vi "EventLogger.Task.FlushToDisk.vi"   [LabVIEW 2019, in "Tools.lvlib"]
uses:
  Tools.lvlib
  EventLogger.Task.FlushToDisk.Action.ctl
  CitTemplate/citTemplate.errData.ctl
types:
  T1 = typedef "Tools.lvlib/citTemplate.errData.ctl" = cluster{"action":string, "error":errorcluster}
  T2 = typedef "Tools.lvlib/EventLogger.Task.FlushToDisk.Action.ctl" = enum32{"idle", "constructor", "destructor", "--- EventLogger.Task.FlushToDisk ---"}
  T3 = typedef "Tools.lvlib/citTemplate.notifierHandle.ctl" = refnum<notifier>
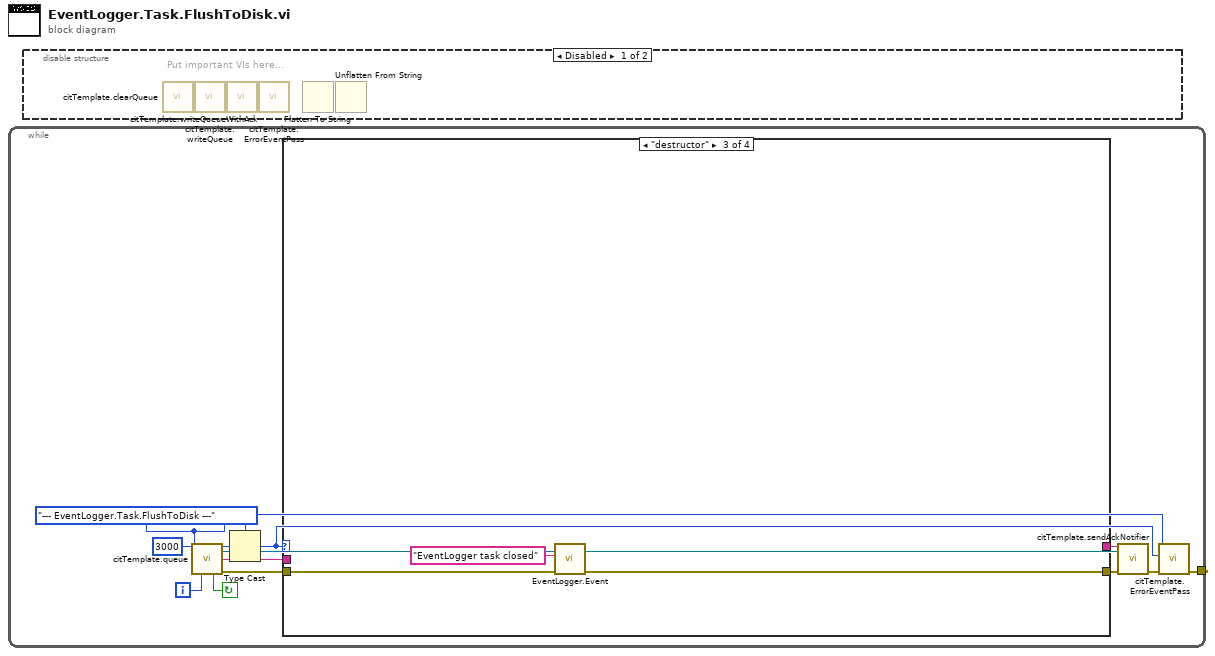
[diagram p0: block diagram]
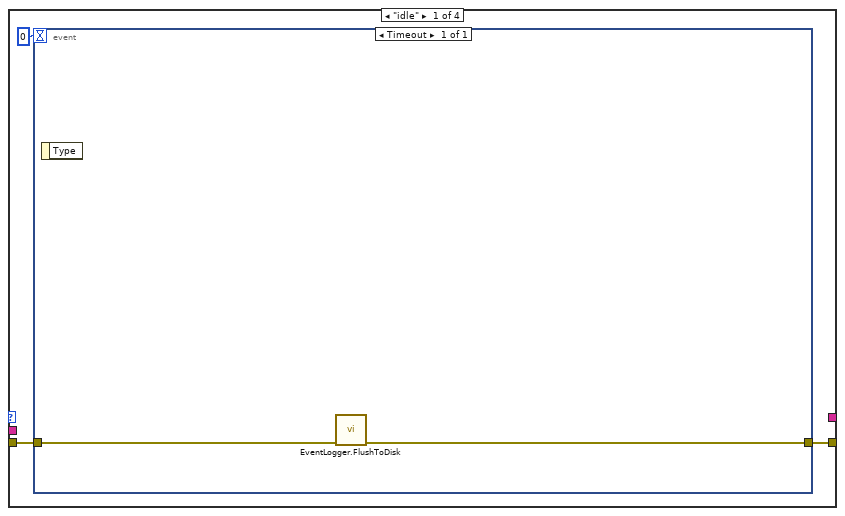
[diagram p3: hidden frame]
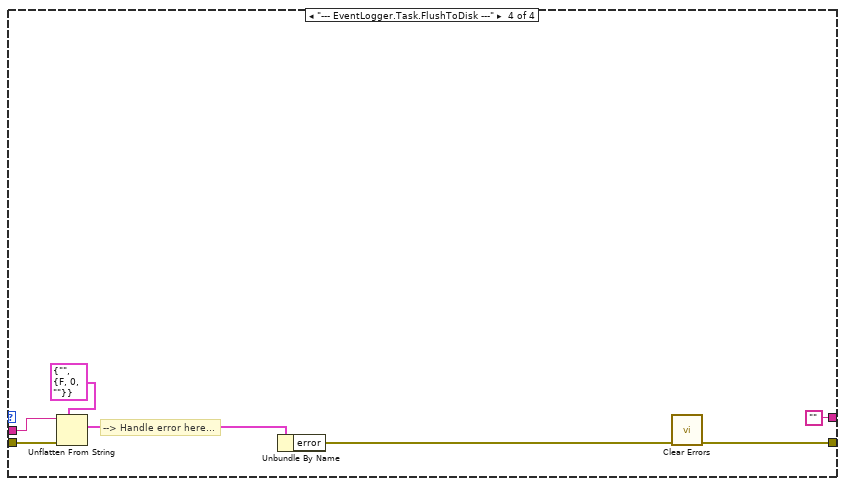
[diagram p5: hidden frame]
diagram:
  n1 = while {
    tunnel: [w2] -> _
    i -> [w8]
    stop <- w9 continue-if-true
    w1 = EventLogger.Task.FlushToDisk.Action."--- EventLogger.Task.FlushToDisk ---" ("Action")
    n2 = call "citTemplate.queue.vi"("ms timeout (250 ms)"=3000, "event enum"=w1, "iteration (-1)"=w8) -> ("notifierHandle out"=w6:T3, "event out"=w12:u32, "(flatten) data out"=w11:string, "continue"=w9:bool, "error out"=w10:errorcluster)  [unwired: 2 in, 6 out]
    n3 = Type Cast(type=w1, x=w12) -> (*(type *) &x=w3:T2)
    n4 = case shown="\"destructor\"" w3 {
      tunnel: w11 -> [_ _ _ w28]
      tunnel: w10 -> [w14 w18 w21 w27]
      tunnel: [w13 w18 w19 w25] -> w4
      tunnel: [_ _ _ ""] -> w5
      frame "idle" {
        n5 = event shown="[0] Timeout" {
          selector: _ -> [_]
          dyn-events: _ -> [_]
          timeout: 0 -> [_]
          tunnel: [w16] -> w13
          tunnel: w14 -> [w17]
          event Timeout {
            n6 = event-data() -> ()  [unwired: 1 in, 1 out]
            n7 = call "EventLogger.FlushToDisk.vi"("error in"=w17) -> ("error out"=w16:errorcluster)  [unwired: 10 in]
          }
        }
      }
      frame "constructor" {
      }
      frame "destructor" {
        n8 = call "EventLogger.Event.vi"("error in"=w21, "Event Name"="EventLogger task closed") -> ("error out"=w19:errorcluster)  [unwired: 9 in]
      }
      frame "--- EventLogger.Task.FlushToDisk ---" {
        # "--> Handle error here..."
        n9 = Unflatten From String(type=T1 {"action"="", "error"={"status"=FALSE, "code"=0, "source"=""}} ("ErrData"), binary string=w28, error in (no error)=w27) -> (value=w26:T1)  [unwired: 4 out]
        n10 = Unbundle By Name(w26) -> ("error"=w22:errorcluster)
        n11 = call <vilib>:"Clear Errors.vi"("error in (no error)"=w22) -> ("error out"=w25:errorcluster)  [unwired: 5 in, 1 out]
      }
    }
    n12 = call "citTemplate.sendAckNotifier.vi"("notification data"=w5, "notifierHandle in"=w6, "error in"=w4) -> ()  [unwired: 13 in]
    n13 = call "citTemplate.ErrorEventPass.vi"("error in (no error)"=w4, "action of error"=w3, "event in"=w1) -> ("error out"=w2:errorcluster)  [unwired: 8 in]
  }
  n14 = disable-structure shown="Disabled" {
    frame Disabled {
      # "Put important VIs here..."
      n15 = call "citTemplate.clearQueue.vi"() -> ()  [unwired: 14 in, 2 out]
      n16 = call "citTemplate.writeQueue.vi"() -> ()  [unwired: 15 in, 1 out]
      n17 = call "citTemplate.writeQueueWithAck.vi"() -> ()  [unwired: 13 in, 3 out]
      n18 = call "citTemplate.ErrorEventPass.vi"() -> ()  [unwired: 11 in, 1 out]
      n19 = Flatten To String() -> ()  [unwired: 4 in, 3 out]
      n20 = Unflatten From String() -> ()  [unwired: 5 in, 3 out]
    }
    frame Enabled {
    }
  }
